vi "Begin.vi"(8 "error in":errorcluster) -> (0 "error out":errorcluster)   [LabVIEW 2019]
doc: "Called before other user functions, this VI is expected to open initial I/O refnums, load in file data, and do all program initialization. Notice that the <B>error out</B> terminal is simply used for data flow. Wiring it to other structures or subVIs ensures that this VI runs first."
uses:
  Robot Global Data.vi
  <vilib>/Rock Robotics/WPI/DriverStation/WPI_DriverStationRobotMode2.ctl
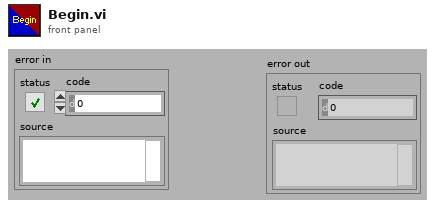
[diagram p1: front panel]
types:
  T1 = typedef "WPI_DriverStationRobotMode2.ctl" = enum16{"Autonomous Disabled", "Autonomous Enabled", "Teleop Disabled", "Teleop Enabled", "Disconnected", "Finish", "Test Disabled", "Test Enabled", "Emergency Stopped"}
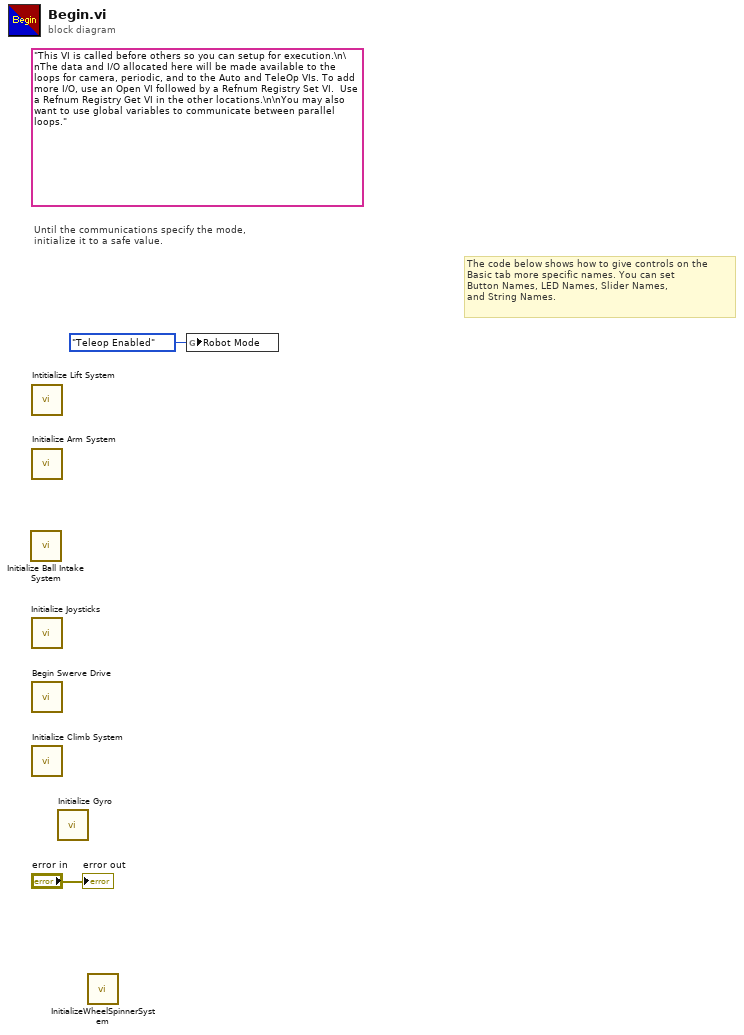
[diagram p0: block diagram]
diagram:
  (unwired) "This VI is called before others so you can setup for execution.\n\nThe data and I/O allocated here will be made available to the loops for camera, periodic, and to the Auto and TeleOp VIs. To add more I/O, use an Open VI followed by a Refnum Registry Set VI.  Use a Refnum Registry Get VI in the other locations.\n\nYou may also want to use global variables to communicate between parallel loops."
  # "The code below shows how to give controls on the\nBasic tab more specific names. You can set\nButton Names, LED Names, Slider Names,\nand String Names."
  # "Until the communications specify the mode,\ninitialize it to a safe value."
  n1 = call "Initialize Ball Intake System.vi"() -> ()  [unwired: 12 in]
  n2 = call "Intitialize Lift System.vi"() -> ()  [unwired: 12 in]
  n3 = call "Initialize Arm System.vi"() -> ()  [unwired: 12 in]
  n4 = call "Initialize Joysticks.vi"() -> ()  [unwired: 12 in]
  n5 = call "Begin Swerve Drive.vi"() -> ()  [unwired: 12 in]
  n6 = call "Initialize Climb System.vi"() -> ()  [unwired: 12 in]
  n7 = call "Initialize Gyro.vi"() -> ()  [unwired: 1 in]
  n8 = call "InitializeWheelSpinnerSystem.vi"() -> ()  [unwired: 12 in]
  n9 = global write "Robot Global Data.vi" "Robot Mode"(WPI_DriverStationRobotMode2."Teleop Enabled" ("Robot Mode")) -> ()
  "error out" <- "error in"
